vi "DAQ.44xx.Get Export Triggers.vi"(8 "error in (no error)":errorcluster, 10 "master task in":refnum<k21>, 11 "task in":refnum<k21>) -> (0 "error out":errorcluster, 3 "task out":refnum<k21>)   [LabVIEW 2019, in "Instrument.DAQ.lvclass"]
uses:
  Instrument.DAQ.lvclass
  <vilib>/DAQmx/configure/trigger.llb/DAQmx Start Trigger (Digital Edge).vi
  <resource>/objmgr/daqmx.rc
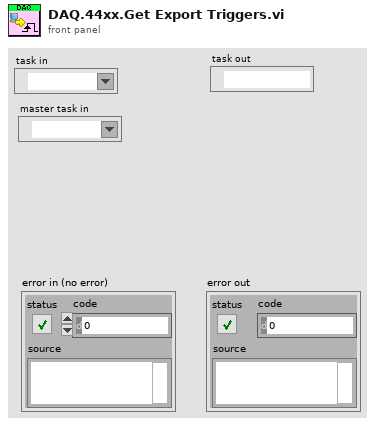
[diagram p1: front panel]
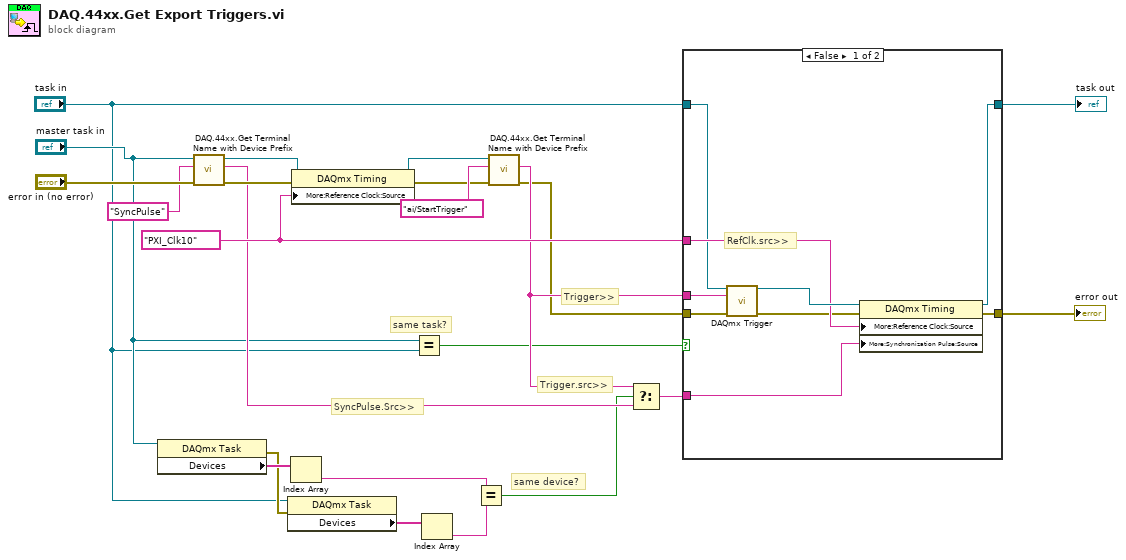
[diagram p0: block diagram]
diagram:
  w15 = tag "PXI_Clk10" ("RefClk.Src")
  # "same task?"
  # "SyncPulse.Src>>"
  # "same device?"
  # "Trigger>>"
  # "Trigger.src>>"
  n1 = property class="DAQmx Task"(reference="master task in") -> (error out=w8:errorcluster, "Devices"=w17:tag[])  [unwired: 1 in, 1 out]
  n2 = call "DAQ.44xx.Get Terminal Name with Device Prefix.vi"("error in (no error)"="error in (no error)", "Local Terminal Name"="SyncPulse", "task/channels in"="master task in") -> ("error out"=w20:errorcluster, "Terminal Name with Device Prefix"=w13:tag, "task out"=w2:refnum<k21>)  [unwired: 6 in]
  n3 = property class="DAQmx Task"(reference="task in", error in=w8) -> ("Devices"=w16:tag[])  [unwired: 2 out]
  n4 = Index Array(array=w17) -> (element=w12:tag)  [unwired: 1 in]
  n5 = property class="DAQmx Timing"(reference=w2, error in=w20, "More:Reference Clock:Source"=w15) -> (reference out=w1:refnum<k21>, error out=w21:errorcluster)
  n6 = Equal?(x="master task in", y="task in") -> (x = y?=w3:bool)
  n7 = Index Array(array=w16) -> (element=w11:tag)  [unwired: 1 in]
  n8 = Equal?(x=w12, y=w11) -> (x = y?=w10:bool)
  n9 = call "DAQ.44xx.Get Terminal Name with Device Prefix.vi"("error in (no error)"=w21, "Local Terminal Name"="ai/StartTrigger", "task/channels in"=w1) -> ("error out"=w9:errorcluster, "Terminal Name with Device Prefix"=w14:tag)  [unwired: 6 in, 1 out]
  n10 = Select(t=w14, s=w10, f=w13) -> (s? t:f=w18:tag)
  n11 = case shown="False" w3 {
    tunnel: w18 -> [w31 _]
    tunnel: w15 -> [w30 _]
    tunnel: w14 -> [w29 _]
    tunnel: w9 -> [w28 w33]
    tunnel: [w27 w34] -> w7
    tunnel: [w25 w33] -> w6
    tunnel: "task in" -> [w24 w34]
    frame False {
      # "RefClk.src>>"
      n12 = call-poly <vilib>:"DAQmx Trigger.vi"("task/channels in"=w24, "source"=w29, "error in"=w28) -> ("task out"=w32:refnum<k21>, "error out"=w26:errorcluster)  [unwired: 11 in]
      n13 = property class="DAQmx Timing"(reference=w32, error in=w26, "More:Reference Clock:Source"=w30, "More:Synchronization Pulse:Source"=w31) -> (reference out=w27:refnum<k21>, error out=w25:errorcluster)
    }
    frame True {
    }
  }
  "error out" <- w6
  "task out" <- w7
